vi "Material-LoadSheet-Dialog.vi"(8 "error in":errorcluster, 11 "Material-RunTest.lvclass in":refnum<class "Material-RunTest.lvclass">) -> (0 "error out":errorcluster, 2 "Cancel Test":bool, 3 "Material-RunTest.lvclass out":refnum<class "Material-RunTest.lvclass">)   [LabVIEW 2014, in "Material-RunTest.lvclass"]
uses:
  Material-RunTest.lvclass
  Motion Control/Motion-ControlAll.lvclass
  Reuse Library/Keyence LK-G5000/Keyence LK-G5000.lvlib
panel:
  in  "Zero Laser":bool
  in  "Apply Vacuum":bool
  in  "Cancel Test":bool
  in  "Help Button":bool
  in  "Last Sheet in lot":bool
  in  "Continue":bool
  out "String":string="Place the sheet of Material on the chuck now. Press the Vacuum button once the sheet is correctly placed on the chuck. Once the sheet if firmly \"Vacuumed\" down press the Continue or Last Sheet button."
  # "Optional"
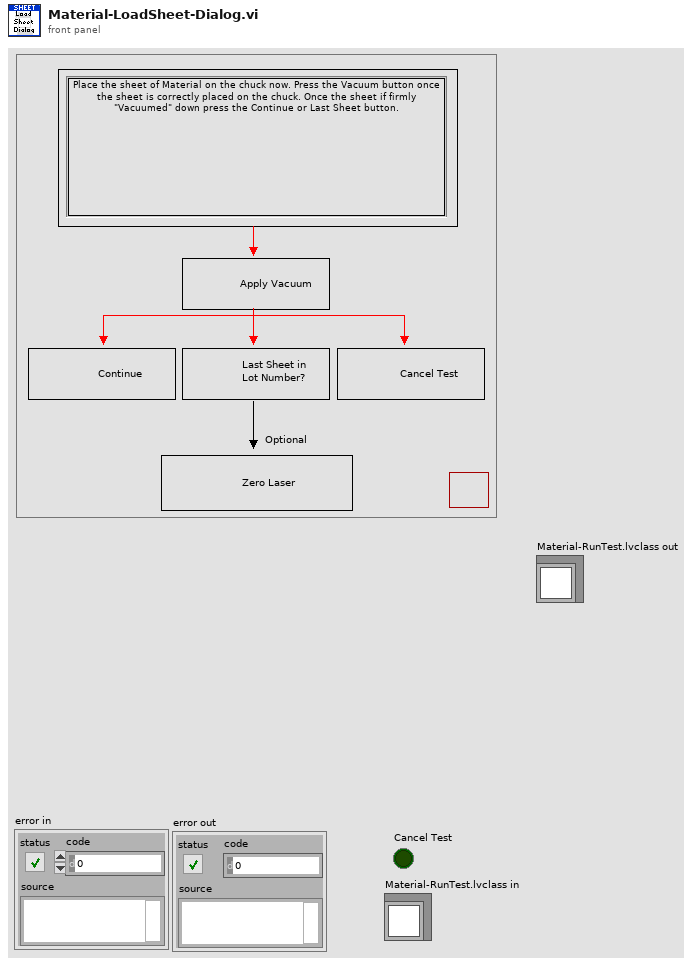
[diagram p1: front panel]
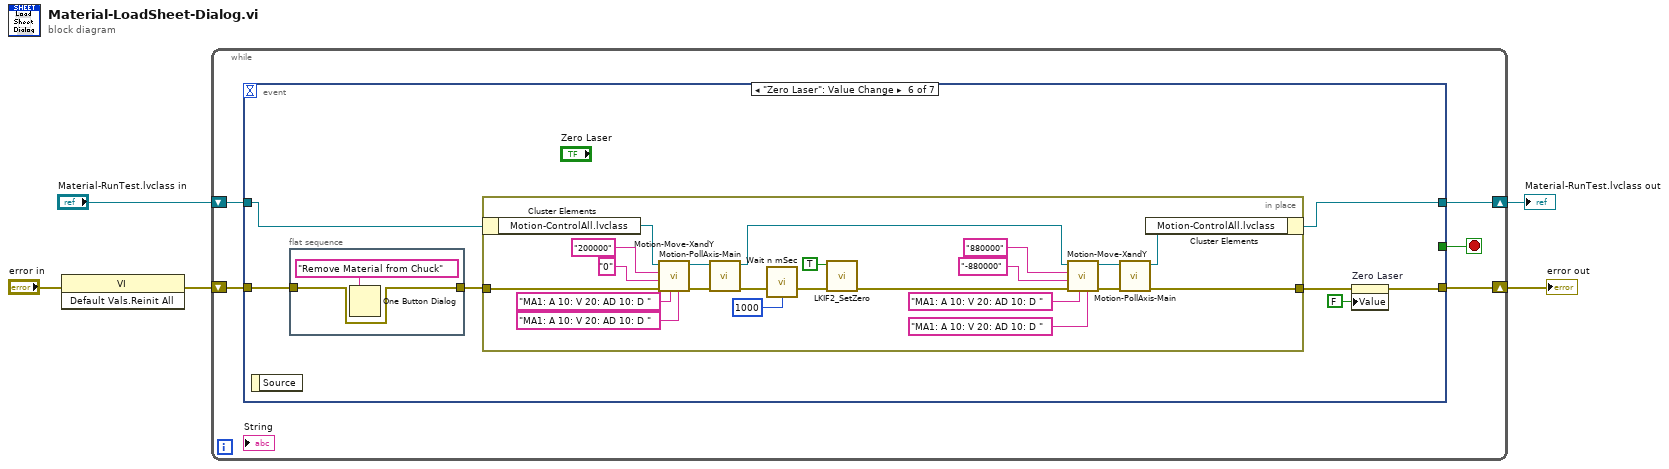
[diagram p0: block diagram]
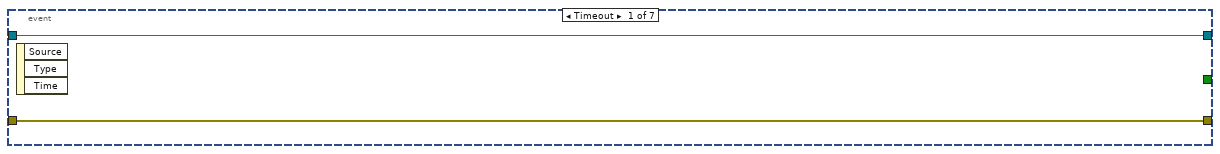
[diagram p2: hidden frame]
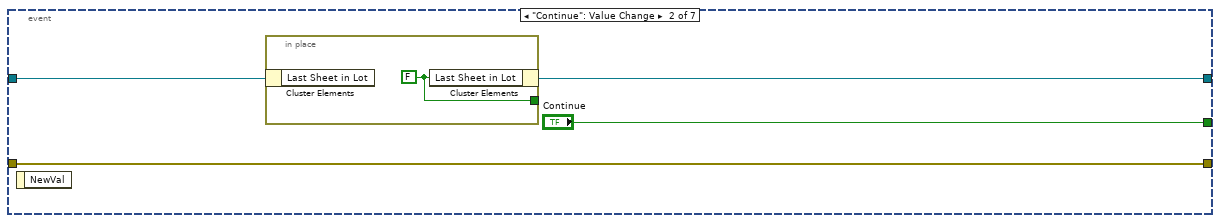
[diagram p3: hidden frame]
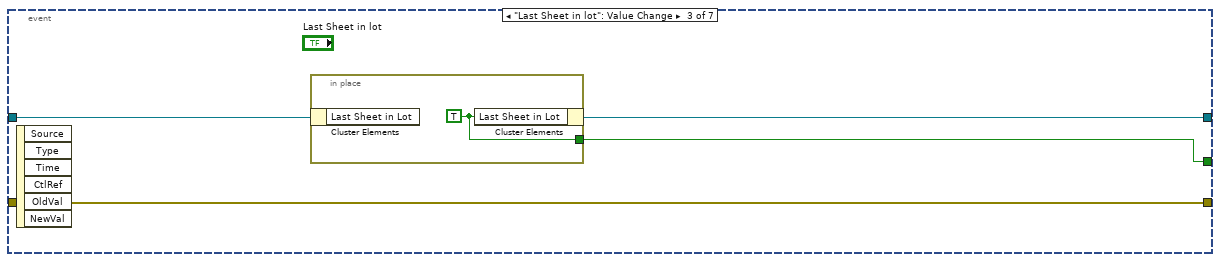
[diagram p4: hidden frame]
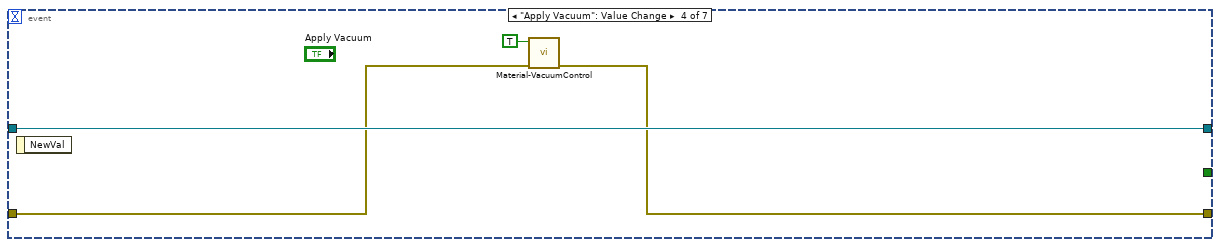
[diagram p5: hidden frame]
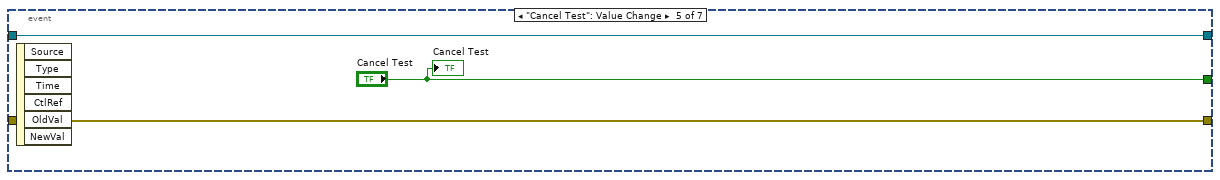
[diagram p6: hidden frame]
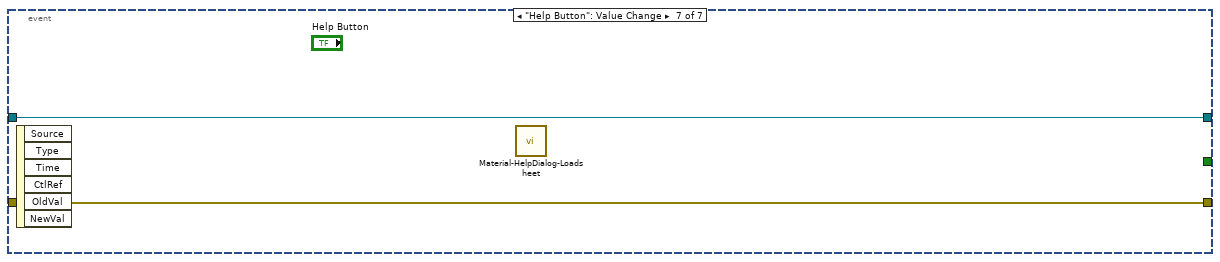
[diagram p7: hidden frame]
diagram:
  n1 = invoke class="VI" method="Default Vals.Reinit All"(error in="error in") -> (error out=w1:errorcluster)  [unwired: 2 in, 2 out]
  n2 = while {
    shift-right: [w8] -> w4
    shift-left: "Material-RunTest.lvclass in" -> [w9]
    shift-right: [w6] -> w3
    shift-left: w1 -> [w7]
    stop <- w10 stop-if-true
    n3 = event shown="[5] \"Zero Laser\": Value Change" {
      selector: _ -> [_ _ _ _ _ _ _]
      dyn-events: _ -> [_ _ _ _ _ _ _]
      timeout: _ -> [_ _ _ _ _ _ _]
      tunnel: [_ "Continue" w19 _ "Cancel Test" _ _] -> w10
      tunnel: w9 -> [w12 w14 w21 w26 w29 w36 w62]
      tunnel: [w12 w13 w20 w26 w29 w35 w62] -> w8
      tunnel: w7 -> [w11 w15 w18 w24 w27 w34 w61]
      tunnel: [w11 w15 w18 w23 w27 w30 w61] -> w6
      event Timeout {
        n4 = event-data() -> ()  [unwired: 1 in, 3 out]
      }
      event "Continue": Value Change {
        n5 = event-data() -> ()  [unwired: 1 in, 1 out]
        n6 = in-place {
          in-place-border: [w17] -> _
          w17 = FALSE ("Last Sheet in Lot")
          n7 = in-place-cluster #1(w14) -> ()  [unwired: 1 out]
          n8 = in-place-cluster #1("Last Sheet in Lot"=w17) -> (w13:refnum<class "Material-RunTest.lvclass">)
        }
      }
      event "Last Sheet in lot": Value Change {
        n9 = event-data() -> ()  [unwired: 1 in, 6 out]
        n10 = in-place {
          in-place-border: [w22] -> w19
          w22 = TRUE ("Last Sheet in Lot")
          n11 = in-place-cluster #2(w21) -> ()  [unwired: 1 out]
          n12 = in-place-cluster #2("Last Sheet in Lot"=w22) -> (w20:refnum<class "Material-RunTest.lvclass">)
        }
      }
      event "Apply Vacuum": Value Change {
        n13 = event-data() -> ()  [unwired: 1 in, 1 out]
        n14 = call "Material-VacuumControl.vi"("error in (no error)"=w24, "Vacuum On/Off"=TRUE) -> ("error out"=w23:errorcluster)  [unwired: 9 in]
      }
      event "Cancel Test": Value Change {
        n15 = event-data() -> ()  [unwired: 1 in, 6 out]
        "Cancel Test" <- "Cancel Test"
      }
      event "Zero Laser": Value Change {
        n16 = event-data() -> ()  [unwired: 1 in, 1 out]
        n17 = flat-sequence {
          tunnel: w34 -> [w37]
          tunnel: [w37] -> w33
          frame #0 {
            n18 = One Button Dialog(message="Remove Material from Chuck") -> ()  [unwired: 1 in, 1 out]
          }
        }
        n19 = in-place {
          in-place-border: w33 -> [w60]
          in-place-border: [w40] -> w32
          n20 = in-place-cluster #3(w36) -> ("Motion-ControlAll.lvclass"=w59:refnum<class "Motion-ControlAll.lvclass">)
          n21 = call "Motion-Move-XandY.vi"("Y Drive Acc/Speed/Velocity"="MA1: A 10: V 20: AD 10: D ", "X Drive Acc/Speed/Velocity"="MA1: A 10: V 20: AD 10: D ", "error in (no error)"=w60, "X Coordinates"="0", "Y Coordinates"="200000", "Motion-ControlAll in"=w59) -> ("error out"=w57:errorcluster, "Motion-ControlAll out"=w58:refnum<class "Motion-ControlAll.lvclass">)  [unwired: 4 in]
          n22 = call "Motion-PollAxis-Main.vi"("error in (no error)"=w57, "Motion-ControlAll in"=w58) -> ("error out"=w52:errorcluster, "Motion-ControlAll out"=w42:refnum<class "Motion-ControlAll.lvclass">)  [unwired: 8 in]
          n23 = call <vilib>:"Wait n mSec.vi"("error in (no error)"=w52, "Milliseconds to Wait (500)"=u32 1000) -> ("error out"=w51:errorcluster)  [unwired: 13 in]
          n24 = call "LKIF2_SetZero.vi"("error in (no error)"=w51, "OnOff"=TRUE) -> ("error out"=w43:errorcluster)  [unwired: 9 in]
          n25 = call "Motion-Move-XandY.vi"("Y Drive Acc/Speed/Velocity"="MA1: A 10: V 20: AD 10: D ", "X Drive Acc/Speed/Velocity"="MA1: A 10: V 20: AD 10: D ", "error in (no error)"=w43, "X Coordinates"="-880000", "Y Coordinates"="880000", "Motion-ControlAll in"=w42) -> ("error out"=w45:errorcluster, "Motion-ControlAll out"=w44:refnum<class "Motion-ControlAll.lvclass">)  [unwired: 4 in]
          n26 = call "Motion-PollAxis-Main.vi"("error in (no error)"=w45, "Motion-ControlAll in"=w44) -> ("error out"=w40:errorcluster, "Motion-ControlAll out"=w41:refnum<class "Motion-ControlAll.lvclass">)  [unwired: 8 in]
          n27 = in-place-cluster #3("Motion-ControlAll.lvclass"=w41) -> (w35:refnum<class "Material-RunTest.lvclass">)
        }
        n28 = property on="Zero Laser" class="Bool (strict)"(error in=w32, "Value"=FALSE ("Zero Laser")) -> (error out=w30:errorcluster)  [unwired: 1 in, 1 out]
      }
      event "Help Button": Value Change {
        n29 = event-data() -> ()  [unwired: 1 in, 6 out]
        n30 = call "Material-HelpDialog-Loadsheet.vi"() -> ()  [unwired: 12 in]
      }
    }
  }
  "error out" <- w3
  "Material-RunTest.lvclass out" <- w4
